vi "Read Motor Controller IDs.vi"(8 "error in (no error)":errorcluster, 10 "settings in":variant, 11 "Tank Drive in":refnum<class "Tank Drive.lvclass">) -> (0 "error out":errorcluster, 3 "Tank Drive out":refnum<class "Tank Drive.lvclass">)   [LabVIEW 2019, in "Drive.lvlib" / "Tank Drive.lvclass"]
uses:
  Tank Drive.lvclass
  Controls/Motor Controller IDs.ctl
  Tank Drive.lvclass/Tank Drive.ctl
  00be1c54-a4dc-4847-a327-bb4ac6293fe5.vi
  05f41a94-2680-4179-a861-3aa4db70521c.vi
  49e0f963-c9a5-4071-8b27-049bfe7eec2a.vi
  9c702a5a-9c9a-4d9a-802b-b3fc84dbf60b.vi
  <vilib>/Utility/error.llb/Trim Whitespace.vi
  <vilib>/Utility/error.llb/Error Cluster From Error Code.vi
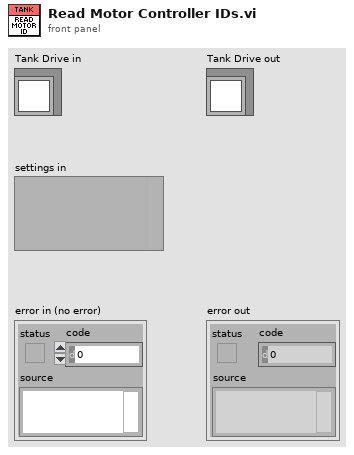
[diagram p1: front panel]
types:
  T1 = typedef "Drive.lvlib/Tank Drive.lvclass/Motor Controller IDs.ctl" = cluster{"Left Lead":u8, "Right Lead":u8, "Left Followers":u8[], "Right Followers":u8[]}
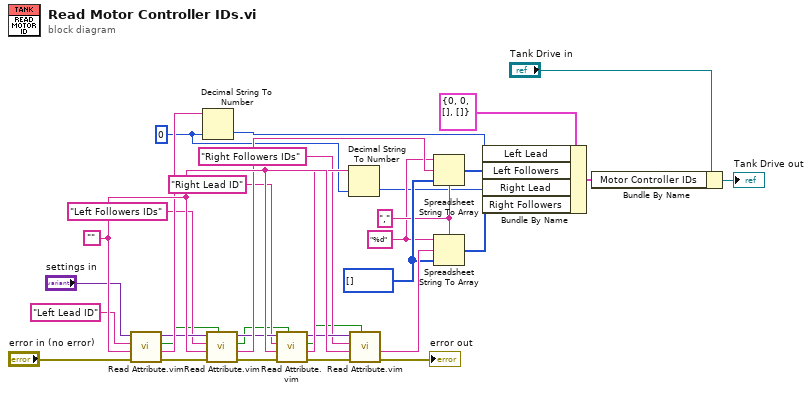
[diagram p0: block diagram]
diagram:
  w1 = u8 0 ("default (0 I32)")
  w17 = u8[] []
  w16 = "," ("delimiter (Tab)")
  w15 = "%d" ("format string")
  w32 = ""
  n1 = call "Read Attribute.vim"("error in"="error in (no error)", "default value (data type)"=w32, "name"="Left Lead ID", "variant in"="settings in") -> ("error out"=w26:errorcluster, "value"=w31:string, "found"=w13:bool, "variant out"=w27:variant)  [unwired: 4 in]
  n2 = Decimal String To Number(string=w31, default (0L)=w1) -> (number=w5:u8)  [unwired: 1 in, 1 out]
  n3 = call "Read Attribute.vim"("Error if not found (T)"=w13, "error in"=w26, "default value (data type)"=w32, "name"="Left Followers IDs", "variant in"=w27) -> ("error out"=w24:errorcluster, "value"=w29:string, "found"=w12:bool, "variant out"=w25:variant)  [unwired: 3 in]
  n4 = call "Read Attribute.vim"("Error if not found (T)"=w12, "error in"=w24, "default value (data type)"=w32, "name"="Right Lead ID", "variant in"=w25) -> ("error out"=w22:errorcluster, "value"=w30:string, "found"=w11:bool, "variant out"=w23:variant)  [unwired: 3 in]
  n5 = Decimal String To Number(string=w30, default (0L)=w1) -> (number=w3:u8)  [unwired: 1 in, 1 out]
  n6 = call "Read Attribute.vim"("Error if not found (T)"=w11, "error in"=w22, "default value (data type)"=w32, "name"="Right Followers IDs", "variant in"=w23) -> ("error out"=→"error out":errorcluster, "value"=w28:string)  [unwired: 3 in, 2 out]
  n7 = Spreadsheet String To Array(delimiter (Tab)=w16, format string=w15, spreadsheet string=w29, array type (2D Dbl)=w17) -> (array=w4:u8[])
  n8 = Spreadsheet String To Array(delimiter (Tab)=w16, format string=w15, spreadsheet string=w28, array type (2D Dbl)=w17) -> (array=w2:u8[])
  n9 = Bundle By Name(cluster=T1 {"Left Lead"=0, "Right Lead"=0, "Left Followers"=[], "Right Followers"=[]} ("Motor Controller IDs"), "Left Lead"=w5, "Left Followers"=w4, "Right Lead"=w3, "Right Followers"=w2) -> (w6:T1)
  n10 = Bundle By Name(cluster="Tank Drive in", "Motor Controller IDs"=w6) -> (→"Tank Drive out":refnum<class "Tank Drive.lvclass">)
